vi "DefaultEscape.vi"() -> (3 "EscapePattern":T1)   [LabVIEW 2009]
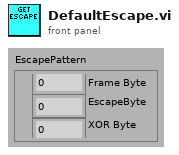
[diagram p1: front panel]
types:
  T1 = cluster{"Frame Byte":u8, "EscapeByte":u8, "XOR Byte":u8}
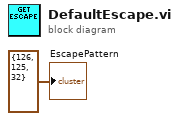
[diagram p0: block diagram]
diagram:
  "EscapePattern" <- T1 {"Frame Byte"=126, "EscapeByte"=125, "XOR Byte"=32} ("input cluster")
